vi "Parse Request.vi"(8 "error in (no error)":errorcluster, 10 "{JSON} Request":string, 11 "JSON-RPC in":refnum<class "JSON-RPC.lvclass">) -> (0 "error out":errorcluster, 1 "Params":string, 2 "Method":string, 3 "JSON-RPC out":refnum<class "JSON-RPC.lvclass">, 4 "ID":string)   [LabVIEW 2019, in "JSON-RPC.lvclass"]
uses:
  JSON-RPC.lvclass
  JSON-RPC.lvclass/JSON-RPC.ctl
  private/Parse Request-JSONtext.vi/523bbeac-5bfa-4355-a479-ec0e355c2dae.vi
  private/Parse Request-JSONtext.vi/5dfc14ef-dff6-4e36-b5f1-09fb62becacc.vi
  private/Parse Request-JSONtext.vi/f339b867-7010-45a6-b71e-b2a9da4366e1.vi
  <vilib>/JDP Science/JSONtext/Find Item.vi
  <vilib>/JDP Science/JSONtext/Next JSON Value.vi
  <vilib>/JDP Science/JSONtext/String Subset.vi
  <vilib>/JDP Science/JSONtext/Parsing/Advance past next JSON Value (inlined COPY).vi
  <vilib>/JDP Science/JSONtext/Parsing/Advance past whitespace.vi
  <vilib>/JDP Science/JSONtext/Parsing/Advance past String.vi
  <vilib>/JDP Science/JSONtext/Parsing/Advance past Number.vi
  <vilib>/JDP Science/JSONtext/Parsing/Advance past Line Ending.vi
  <vilib>/JDP Science/JSONtext/Get all Object Items.vi
  <vilib>/JDP Science/JSONtext/Parsing/Parse Full Path or Item Name.vi
  <vilib>/JDP Science/JSONtext/Parsing/Advance past Array.vi
  <vilib>/JDP Science/JSONtext/Parsing/Advance past Object.vi
  <vilib>/JDP Science/JSONtext/support/Error Cluster From Code.vi
  <vilib>/JDP Science/JSONtext/Offset/Find Item Locations by Path.vi
  <vilib>/JDP Science/JSONtext/JSON text to Variant.vi
  <vilib>/JDP Science/JSONtext/LVClass Serializer/JSONtext LVClass Serializer.lvclass
  <vilib>/JDP Science/JSONtext/JSONtext.lvlib
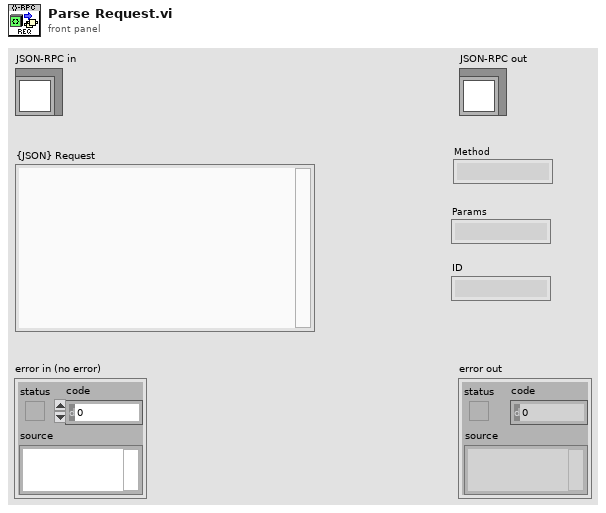
[diagram p1: front panel]
types:
  T1 = typedef "JSONtext.lvlib/JSON Value Type.ctl" = enum16{"Not a JSON Value", "JSON Object", "JSON Array", "String", "Number", "true", "false", "null"}
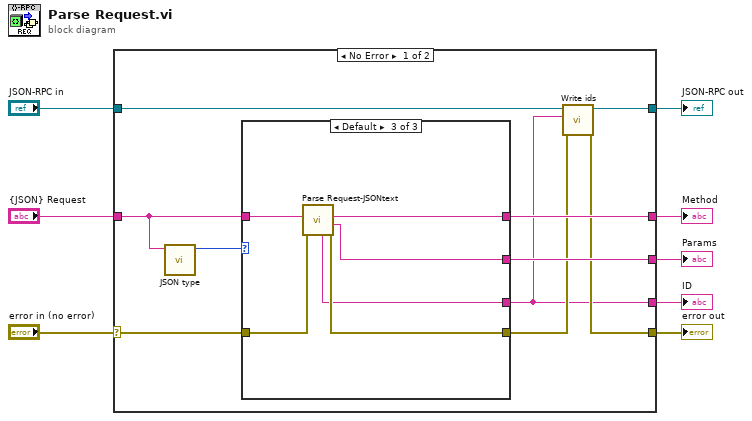
[diagram p0: block diagram]
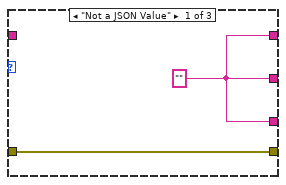
[diagram p2: hidden frame]
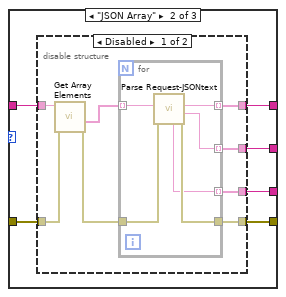
[diagram p3: hidden frame]
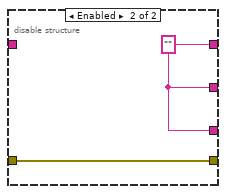
[diagram p4: hidden frame]
diagram:
  n1 = case shown="No Error" "error in (no error)" {
    selector: "error in (no error)" -> [w15 w50]
    tunnel: [w12 w50] -> w7
    tunnel: [w11 w49] -> w5
    tunnel: "JSON-RPC in" -> [w10 w49]
    tunnel: "{JSON} Request" -> [w14 _]
    tunnel: [w18 _] -> w2
    tunnel: [w17 _] -> w3
    tunnel: [w9 _] -> w1
    frame No Error {
      n2 = call <vilib>:"JSON type.vi"("JSON"=w14) -> ("JSON Value Type"=w16:T1)  [unwired: 9 in, 1 out]
      n3 = case shown="Default" w16 {
        tunnel: w15 -> [w20 w22 w45]
        tunnel: [w20 w26 w44] -> w13
        tunnel: w14 -> [_ w23 w48]
        tunnel: [w19 w25 w47] -> w17
        tunnel: [w19 w24 w46] -> w18
        tunnel: [w19 w21 w43] -> w9
        frame "Not a JSON Value" {
          w19 = ""
        }
        frame "JSON Array" {
          n4 = disable-structure shown="Disabled" {
            disable-tunnel: [w34 w41] -> w26
            disable-tunnel: [w33 w42] -> w25
            disable-tunnel: [w32 w42] -> w24
            disable-tunnel: w23 -> [w31 _]
            disable-tunnel: w22 -> [w30 w41]
            disable-tunnel: [w28 w42] -> w21
            frame Disabled {
              n5 = call <vilib>:"Get Array Elements.vi"("error in (no error)"=w30, "JSON"=w31) -> ("error out"=w27:errorcluster, "<JSON>"=w29:string[])  [unwired: 7 in, 1 out]
              n6 = for {
                tunnel: w29 -> [w38] mode=indexing
                tunnel: [w37] -> w33 mode=indexing
                tunnel: [w35] -> w32 mode=indexing
                tunnel: [w36] -> w28 mode=indexing
                tunnel: w27 -> [w39]
                tunnel: [w40] -> w34
                n7 = call "Parse Request-JSONtext.vi"("error in (no error)"=w39, "{JSON} Request"=w38) -> ("error out"=w40:errorcluster, "params"=w35:string, "method"=w37:string, "id"=w36:string)  [unwired: 6 in]
              }
            }
            frame Enabled {
              w42 = ""
            }
          }
        }
        frame Default {
          n8 = call "Parse Request-JSONtext.vi"("error in (no error)"=w45, "{JSON} Request"=w48) -> ("error out"=w44:errorcluster, "params"=w46:string, "method"=w47:string, "id"=w43:string)  [unwired: 6 in]
        }
      }
      n9 = call "Write ids.vi"("error in (no error)"=w13, "ids"=w9, "JSON-RPC in"=w10) -> ("error out"=w12:errorcluster, "JSON-RPC out"=w11:refnum<class "JSON-RPC.lvclass">)  [unwired: 7 in]
    }
    frame Error {
    }
  }
  "error out" <- w7
  "JSON-RPC out" <- w5
  "Method" <- w3
  "Params" <- w2
  "ID" <- w1
